vi "filter.ip.vi"(9 "reset":bool, 10 "debug":bool) -> ()   [LabVIEW 2020]
uses:
  builds/fpganow.common/orderbook.command.type.ctl
  <vilib>/Platform/TimedLoop/XDataNode/timing_clust.ctl
  <vilib>/Platform/TimedLoop/XDataNode/nitl_modes.ctl
  <vilib>/Platform/TimedLoop/XDataNode/wakeup.ctl
  ticker.slot.ctl
  builds/fpganow.common/orderbook.command.ctl
  <vilib>/rvi/Emulation/niFpgaSctlEmulationGetInTimedLoop.vi
  <vilib>/rvi/Emulation/niFpgaEmulationReportErrorSimple.vi
  <vilib>/rvi/Emulation/niFpgaGetClockAttributes.vi
  <vilib>/rvi/Emulation/niFpgaCriticalErrorInLSC.vi
  <vilib>/rvi/Emulation/niFpgaEmulationIsFPGAContextNoSignature.vi
  <vilib>/rvi/errors/niFpgaSetErrorForExecOnDevCompSimple.vi
  <vilib>/rvi/eio/common/nirviEmuReportErrorAndStop.vi
  <vilib>/rvi/DataTransferAndStorage/Container/Common/niFpgaContainerGetUniqueNameForEmu.vi
  <vilib>/rvi/FIFO/Fifo_Resource/nirvififoEmulationSetSize.vi
  <vilib>/rvi/FIFO/Fifo_Resource/nirviFifoEmulationQueueMgr.vi
  <instcachedir>/0/nirviFifoEmulationQueueMgr_E5CAEC123FF24DC58D834DCA3CDAA9B5.lvgen/nirviFifoEmulationQueueMgr_E5CAEC123FF24DC58D834DCA3CDAA9B5_001.vi
  <vilib>/Utility/error.llb/Clear Errors.vi
  <vilib>/rvi/FIFO/Fifo_Resource/nirvififoEmulationCreateLock.vi
  <vilib>/rvi/Emulation/niFpgaProcessEmulError.vi
  <vilib>/rvi/FIFO/Fifo_Resource/nirvififoEmulationObtainLock.vi
  <vilib>/rvi/FIFO/Fifo_Resource/nirvififoEmulationReleaseLock.vi
  <vilib>/rvi/occurrence/nirviWaitOnOccurrenceBase.vi
  <vilib>/rvi/errors/nirviReportUnexpectedCaseInternalError.vi
  <vilib>/rvi/errors/nirviReportUnexpectedCaseInternalError (U32).vi
  <instcachedir>/0/nirviFifoEmulationQueueMgr_E5CAEC123FF24DC58D834DCA3CDAA9B5.lvgen/nirviFifoEmulationQueueMgr_E5CAEC123FF24DC58D834DCA3CDAA9B5_000.vi
  <vilib>/rvi/FIFO/Fifo_Resource/nirvififoEmulationDetermineInputValidOut.vi
  <vilib>/rvi/DataTransferAndStorage/Container/Common/niFpgaContainerSetEmuInfo.vi
  <vilib>/rvi/DataTransferAndStorage/Container/Common/niFpgaContainerExecOnDevCompGetState.vi
  <instcachedir>/0/nirviFifoEmulationQueueMgr_E5CAEC123FF24DC58D834DCA3CDAA9B5.lvgen/nirviFifoEmulationQueueMgr_E5CAEC123FF24DC58D834DCA3CDAA9B5_002.vi
  <vilib>/rvi/interface/RandomDataEmulation/niFpgaRandomDataHandleErrors.vi
  <vilib>/Platform/TimedLoop/XDataNode/XDataNode.xnode
  <vilib>/rvi/DataTransferAndStorage/Container/XNode/niFpgaContainer.xnode
  <vilib>/rvi/FIFO/Fifo_Resource/nirvififoEmulationRead.vi
  <vilib>/rvi/FIFO/Fifo_Resource/nirvififoEmulationWrite.vi
  <vilib>/rvi/LocalResourceManager/LocalResourceManager.xnode
  <vilib>/rvi/FIFO/Fifo_Resource/niFpgaFifoEmulationRefIn.vi
  <vilib>/Platform/TimedLoop/XDataNode/XDNodeRunTimeDep.lvlib
  builds/fpganow.common/fpganow.common.fpga.lvlib
panel:
  in  "Command.In.nanoseconds":u64
  in  "Command.In.seconds":u64
  in  "Command.In.remaining.qty":u32
  in  "Command.In.canceled.qty":u32
  in  "Command.In.executed.qty":u32
  in  "Command.In.price":u64
  in  "Command.In.symbol":u64
  in  "Command.In.quantity":u32
  in  "Command.In.orderId":u64
  in  "Command.In.side":u8
  in  "Command.In.type":T1
  out "Command.Out.Remove":bool
  out "Command.Out.Edit":bool
  out "Command.Out.Add":bool
  out "Command.Out.nanoseconds":u64
  out "Command.Out.seconds":u64
  out "Command.Out.remaining.qty":u32
  out "Command.Out.canceled.qty":u32
  out "Command.Out.executed.qty":u32
  out "Command.Out.price":u64
  out "Command.Out.symbol":u64
  out "Command.Out.quantity":u32
  out "Command.Out.orderId":u64
  out "Command.Out.side":u8
  out "Command.Out.type":T2(ring)
  in  "Command.In.Valid":bool
  out "State.Out.Valid":bool
  out "State.Out.Quantity":u64
  out "State.Out.OrderId":u64
  out "Command.Out.Valid":bool
  out "Debug.Data":cluster{"Ticker":u64, "OrderId":u64}
  out "Debug.Valid":bool
  in  "Symbol.Valid":bool
  in  "Symbol":u64
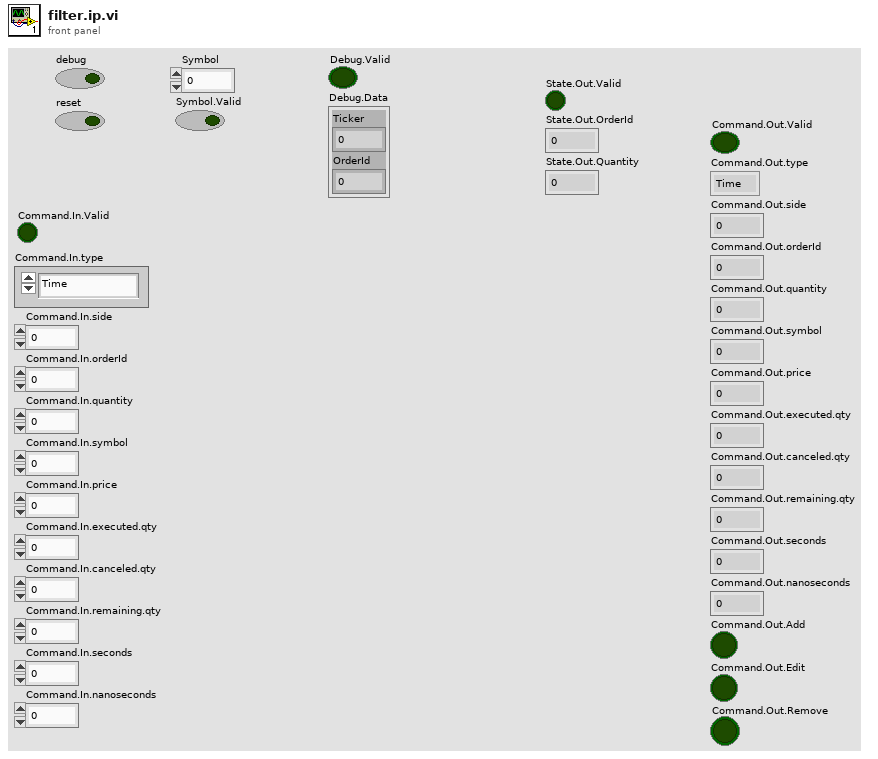
[diagram p1: front panel]
types:
  T1 = typedef "fpganow.common.fpga.lvlib/orderbook.command.type.ctl" = enum8{"Time", "AddOrder", "OrderExecuted", "OrderExecutedAtPrice", "ReduceSize", "ModifyOrder", "DeleteOrder", "Get.Everything", "Get.All.Orders", "Get.Top"}
  T2 = enum8{"Time", "AddOrder", "OrderExecuted", "OrderExecutedAtPrice", "ReduceSize", "ModifyOrder", "DeleteOrder", "Get.Everything", "Get.All.Orders", "Get.Top"}
  T3 = typedef "XDNodeRunTimeDep.lvlib/timing_clust.ctl" = cluster{"Expected End [f-1]":u64, "Actual End [f-1]":u64, "Finished Late? [f-1]":bool, "Expected End [i-1]":u64, "Actual End [i-1]":u64, "Finished Late? [i-1]":bool, "Expected Start [i]":u64, "Actual Start [i]":u64, "Expected Start [f]":u64, "Actual Start [f]":u64, "Source Name":string, "Structure Name":string, "Period":i64, "Deadline":i64, "Offset":i64, "Start":i64, "Priority":i32, "Timeout":i32, "Mode":T4, "Wakeup Reason":T5, "Error":errorcluster, "Source Type":string, "Secondary Source Type":string, "Global End Time":u64, "Global Start Time":u64, "Frame Duration":u64, "Iteration Duration":u64, "Assigned CPU":i32, "I/O Scan Engine Mode":u32}
  T4 = typedef "XDNodeRunTimeDep.lvlib/nitl_modes.ctl" = enum32{"No Change", "Process missed periods, maintain original phase", "Discard missed periods, maintain original phase", "Process missed periods, ignore original phase", "Discard missed periods, ignore original phase"}
  T5 = typedef "XDNodeRunTimeDep.lvlib/wakeup.ctl" = enum32{"Normal", "Aborted", "Asynchronous wakeup", "Timing source error", "Timed loop error", "Timeout"}
  T6 = typedef "fpganow.common.fpga.lvlib/orderbook.command.ctl" = cluster{"type":T1, "side":u8, "orderId ":u64, "quantity":u32, "symbol":u64, "price":u64, "executed.qty":u32, "canceled.qty":u32, "remaining.qty":u32, "seconds":u64, "nanoseconds":u64, "Add":bool, "Edit":bool, "Remove":bool}
  T7 = typedef "ticker.slot.ctl" = cluster{"Symbol":u64}
  T8 = cluster{"type":enum8{"Time", "AddOrder", "OrderExecuted", "OrderExecutedAtPrice", "ReduceSize", "ModifyOrder", "DeleteOrder", "Get.Everything", "Get.All.Orders", "Get.Top"}, "side":u8, "orderId ":u64, "quantity":u32, "symbol":u64, "price":u64, "executed.qty":u32, "canceled.qty":u32, "remaining.qty":u32, "seconds":u64, "nanoseconds":u64, "Add":bool, "Edit":bool, "Remove":bool}
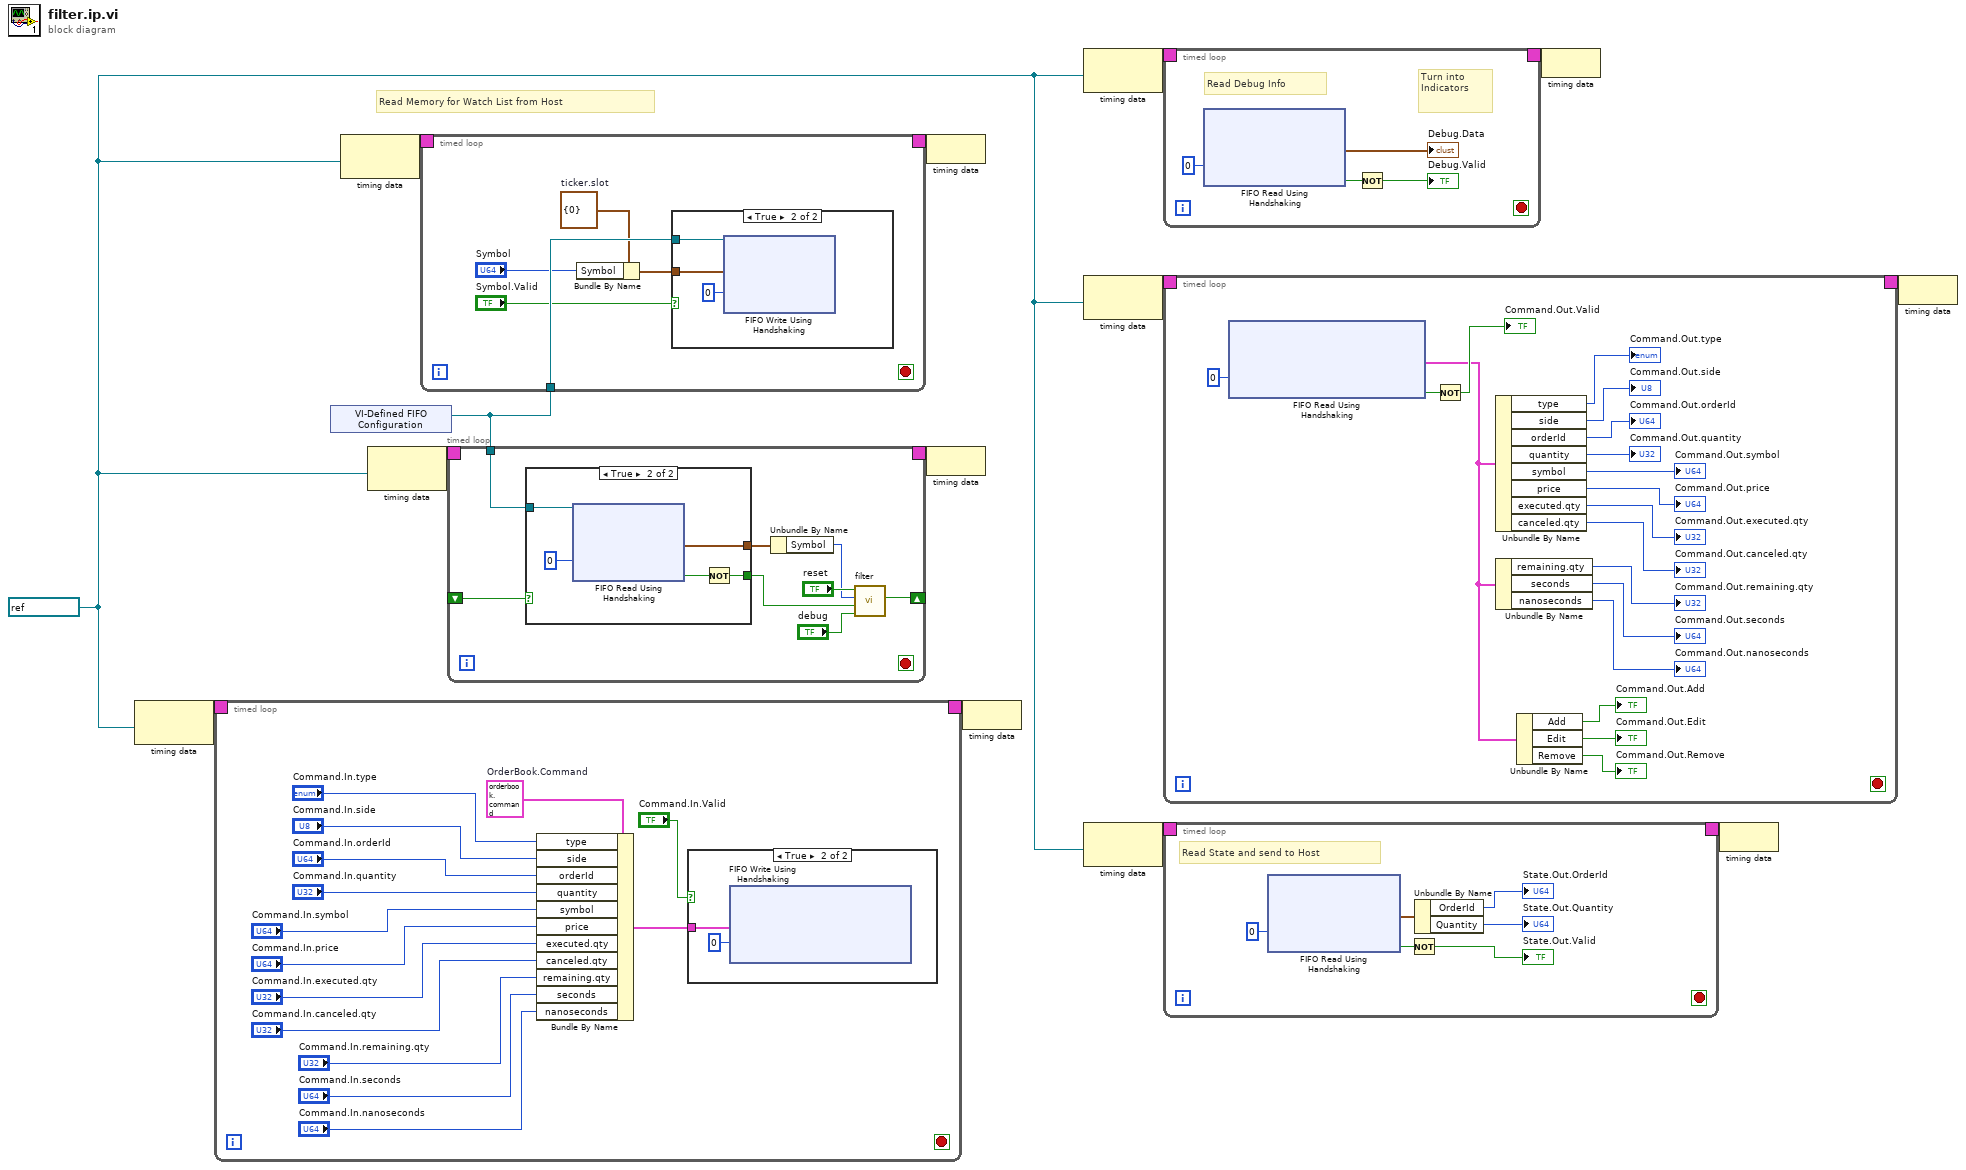
[diagram p0: block diagram]
diagram:
  w1 = refnum<k21> "100MHz" ("Source Name")
  # "Read Memory for Watch List from Host"
  n1 = node-c288(w1) -> (w7:T3)
  n2 = timed-loop {
    timing: w7 -> [_]
    timing-out: [_] -> w6
    stop <- _ stop-if-true
    w28 = T6 {"type"=enum."AddOrder", "side"=0, "orderId "=0, "quantity"=0, "symbol"=0, "price"=0, "executed.qty"=0, "canceled.qty"=0, "remaining.qty"=0, "seconds"=0, "nanoseconds"=0, "Add"=FALSE, "Edit"=FALSE, "Remove"=FALSE}  # OrderBook.Command
    n3 = Bundle By Name(cluster=w28, "type"="Command.In.type", "side"="Command.In.side", "orderId"="Command.In.orderId", "quantity"="Command.In.quantity", "symbol"="Command.In.symbol", "price"="Command.In.price", "executed.qty"="Command.In.executed.qty", "canceled.qty"="Command.In.canceled.qty", "remaining.qty"="Command.In.remaining.qty", "seconds"="Command.In.seconds", "nanoseconds"="Command.In.nanoseconds") -> (w27:T6)
    n4 = case shown="True" "Command.In.Valid" {
      tunnel: w27 -> [_ w30]
      frame False {
      }
      frame True {
        n5 = xnode ("FIFO Write Using Handshaking")("Element"=w30, "Timeout"=0) -> ()  [unwired: 1 in, 2 out]
      }
    }
  }
  n6 = xnode "VI-Defined FIFO Configuration"() -> ("FIFO Out"=w10:refnum<k21>)
  n7 = node-c288(w1) -> (w12:T3)
  n8 = node-c288(w1) -> (w14:T3)
  n9 = timed-loop {
    timing: w12 -> [_]
    timing-out: [_] -> w11
    tunnel: w10 -> [w37]
    stop <- _ stop-if-true
    w36 = T7 {"Symbol"=0}  # ticker.slot
    n10 = Bundle By Name(cluster=w36, "Symbol"="Symbol") -> (w35:T7)
    n11 = case shown="True" "Symbol.Valid" {
      tunnel: w37 -> [_ w40]
      tunnel: w35 -> [_ w39]
      frame False {
      }
      frame True {
        n12 = xnode ("FIFO Write Using Handshaking")("Element"=w39, "Timeout"=0, "FIFO In"=w40) -> ()  [unwired: 2 out]
      }
    }
  }
  n13 = timed-loop {
    timing: w14 -> [_]
    timing-out: [_] -> w13
    tunnel: w10 -> [w50]
    shift-right: [w45] -> _
    shift-left: _ -> [w43]
    stop <- _ stop-if-true
    n14 = case shown="True" w43 {
      tunnel: w50 -> [_ w55]
      tunnel: [_ w54] -> w49
      tunnel: [_ w51] -> w47
      frame False {
      }
      frame True {
        n15 = xnode ("FIFO Read Using Handshaking")("Timeout"=0, "FIFO In"=w55) -> ("Element"=w54:cluster{"Symbol":u64}, "Timed Out?"=w52:bool)  [unwired: 1 out]
        n16 = Not(x=w52) -> (.not. x?=w51:bool)
      }
    }
    n17 = Unbundle By Name(w49) -> ("Symbol"=w44:u64)
    n18 = call "filter.vi"("debug"="debug", "conf.valid"=w47, "conf"=w44, "reset"="reset") -> ("Ready.for.Configuration.Input"=w45:bool)  [unwired: 6 in, 1 out]
  }
  n19 = node-c288(w11) -> ()
  n20 = node-c288(w13) -> ()
  n21 = node-c288(w6) -> ()
  n22 = node-c288(w1) -> (w9:T3)
  n23 = node-c288(w1) -> (w5:T3)
  n24 = node-c288(w1) -> (w3:T3)
  n25 = timed-loop {
    timing: w9 -> [_]
    timing-out: [_] -> w8
    stop <- _ stop-if-true
    # "Turn into \nIndicators"
    # "Read Debug Info"
    n26 = xnode ("FIFO Read Using Handshaking")("Timeout"=0) -> ("Element"=→"Debug.Data":cluster{"Ticker":u64, "OrderId":u64}, "Timed Out?"=w60:bool)  [unwired: 1 in, 1 out]
    n27 = Not(x=w60) -> (.not. x?=→"Debug.Valid":bool)
  }
  n28 = timed-loop {
    timing: w5 -> [_]
    timing-out: [_] -> w4
    stop <- _ stop-if-true
    n29 = xnode ("FIFO Read Using Handshaking")("Timeout"=0) -> ("Element"=w67:T8, "Timed Out?"=w80:bool)  [unwired: 1 in, 1 out]
    n30 = Not(x=w80) -> (.not. x?=→"Command.Out.Valid":bool)
    n31 = Unbundle By Name(w67) -> ("type"=→"Command.Out.type":T2, "side"=→"Command.Out.side":u8, "orderId"=→"Command.Out.orderId":u64, "quantity"=→"Command.Out.quantity":u32, "symbol"=→"Command.Out.symbol":u64, "price"=→"Command.Out.price":u64, "executed.qty"=→"Command.Out.executed.qty":u32, "canceled.qty"=→"Command.Out.canceled.qty":u32)
    n32 = Unbundle By Name(w67) -> ("remaining.qty"=→"Command.Out.remaining.qty":u32, "seconds"=→"Command.Out.seconds":u64, "nanoseconds"=→"Command.Out.nanoseconds":u64)
    n33 = Unbundle By Name(w67) -> ("Add"=→"Command.Out.Add":bool, "Edit"=→"Command.Out.Edit":bool, "Remove"=→"Command.Out.Remove":bool)
  }
  n34 = timed-loop {
    timing: w3 -> [_]
    timing-out: [_] -> w2
    stop <- _ stop-if-true
    # "Read State and send to Host"
    n35 = xnode ("FIFO Read Using Handshaking")("Timeout"=0) -> ("Element"=w89:cluster{"OrderId":u64, "Quantity":u64}, "Timed Out?"=w87:bool)  [unwired: 1 in, 1 out]
    n36 = Not(x=w87) -> (.not. x?=→"State.Out.Valid":bool)
    n37 = Unbundle By Name(w89) -> ("OrderId"=→"State.Out.OrderId":u64, "Quantity"=→"State.Out.Quantity":u64)
  }
  n38 = node-c288(w8) -> ()
  n39 = node-c288(w2) -> ()
  n40 = node-c288(w4) -> ()
